vi "RSZVB Application Example.vi"(0 "VISA session":refnum<visa-resource-name>, 1 "Start Frequency (300.0e3 Hz)":dbl=300000.0 format="%^.3e", 2 "Power (0.0 dBm)":dbl format="%^.3e", 5 "Channel (1)":i32=1, 11 "error in (no error)":errorcluster {"code" format="%.0x"}, 12 "Stop Frequency (4.0e9 Hz)":dbl=4000000000.0 format="%^.3e") -> (4 "dup VISA session":refnum<visa-resource-name>, 6 "Stimulus Data":dbl[](array[numeric]) format="%^.3e", 8 "Response Data":dbl[](array[numeric]) format="%^.3e", 15 "error out":errorcluster {"code" format="%.0x"})   [LabVIEW 2011]
doc: "This VI is an simple example how to use instrument driver VIs."
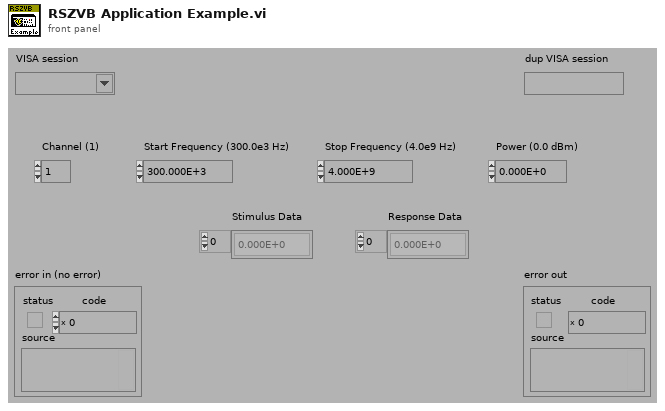
[diagram p1: front panel]
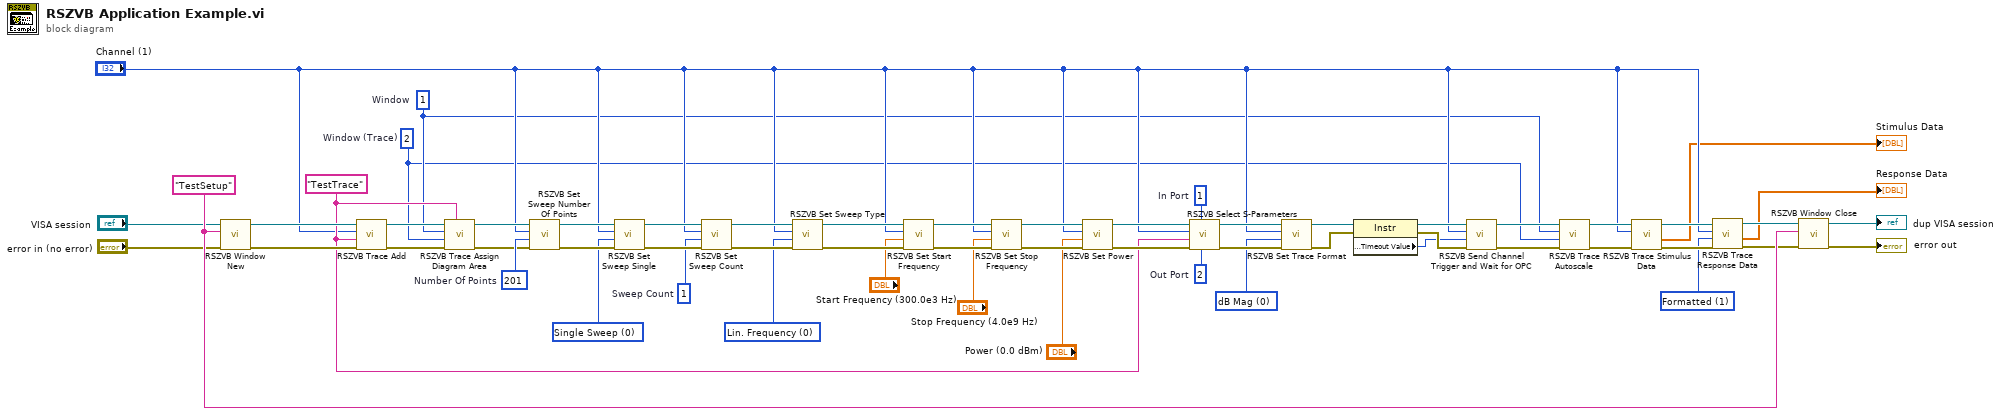
[diagram p0: block diagram]
diagram:
  w25 = 2  # Out Port
  w26 = 1  # In Port
  w6 = 2  # Window (Trace)
  w7 = 1  # Window
  w36 = 0 items=["dB Mag", "Phase", "Smith", "Polar", "Delay", "SWR", "Lin Mag", "Real", "Imag", "Inverted Smith", "Unwrapped Phase"] ("Format (0: dB Mag)")
  w39 = 1 items=["Unformatted", "Formatted"] ("Data Format (0: Unformatted)")
  w46 = 0 items=["Lin. Frequency", "Log. Frequency", "Segmented Frequency", "Power", "Time", "CW Mode"] ("Sweep Type (0: Lin. Frequency)")
  w49 = 201  # Number Of Points
  w50 = 1  # Sweep Count
  w51 = 0 items=["Single Sweep", "Continuous Sweep"] ("Single Sweep (1: Continuous Sweep)")
  w27 = "TestTrace" ("Trace Name (Trc1)")
  w24 = "TestSetup" ("Setup Name (Set1)")
  n1 = call "RSZVB Window New.vi"("error in (no error)"="error in (no error)", "Setup Name (Set1)"=w24, "VISA session"="VISA session") -> ("error out"=w57:errorcluster, "dup VISA session"=w56:refnum<visa-resource-name>)  [unwired: 7 in]
  n2 = call "RSZVB Trace Add.vi"("error in (no error)"=w57, "Trace Name (Trc1)"=w27, "Channel (1)"="Channel (1)", "VISA session"=w56) -> ("error out"=w30:errorcluster, "dup VISA session"=w31:refnum<visa-resource-name>)  [unwired: 6 in]
  n3 = call "RSZVB Trace Assign Diagram Area.vi"("Trace Name (Trc1)"=w27, "error in (no error)"=w30, "Window (Trace) (1)"=w6, "Window (1)"=w7, "VISA session"=w31) -> ("error out"=w28:errorcluster, "dup VISA session"=w29:refnum<visa-resource-name>)  [unwired: 5 in]
  n4 = call "RSZVB Set Sweep Number Of Points.vi"("error in (no error)"=w28, "Number Of Points (201)"=w49, "Channel (1)"="Channel (1)", "VISA session"=w29) -> ("error out"=w54:errorcluster, "dup VISA session"=w55:refnum<visa-resource-name>)  [unwired: 6 in]
  n5 = call "RSZVB Set Sweep Single.vi"("error in (no error)"=w54, "Single Sweep (1: Continuous Sweep)"=w51, "Channel (1)"="Channel (1)", "VISA session"=w55) -> ("error out"=w52:errorcluster, "dup VISA session"=w53:refnum<visa-resource-name>)  [unwired: 6 in]
  n6 = call "RSZVB Set Sweep Count.vi"("error in (no error)"=w52, "Sweep Count (1)"=w50, "Channel (1)"="Channel (1)", "VISA session"=w53) -> ("error out"=w47:errorcluster, "dup VISA session"=w48:refnum<visa-resource-name>)  [unwired: 6 in]
  n7 = call "RSZVB Set Sweep Type.vi"("error in (no error)"=w47, "Sweep Type (0: Lin. Frequency)"=w46, "Channel (1)"="Channel (1)", "VISA session"=w48) -> ("error out"=w44:errorcluster, "dup VISA session"=w45:refnum<visa-resource-name>)  [unwired: 6 in]
  n8 = call "RSZVB Set Start Frequency.vi"("error in (no error)"=w44, "Start Frequency (300.0e3 Hz)"="Start Frequency (300.0e3 Hz)", "Channel (1)"="Channel (1)", "VISA session"=w45) -> ("error out"=w14:errorcluster, "dup VISA session"=w15:refnum<visa-resource-name>)  [unwired: 6 in]
  n9 = call "RSZVB Set Stop Frequency.vi"("error in (no error)"=w14, "Stop Frequency (8.0e9 Hz)"="Stop Frequency (4.0e9 Hz)", "Channel (1)"="Channel (1)", "VISA session"=w15) -> ("error out"=w12:errorcluster, "dup VISA session"=w13:refnum<visa-resource-name>)  [unwired: 6 in]
  n10 = call "RSZVB Set Power.vi"("error in (no error)"=w12, "Power (0.0 dBm)"="Power (0.0 dBm)", "Channel (1)"="Channel (1)", "VISA session"=w13) -> ("error out"=w42:errorcluster, "dup VISA session"=w43:refnum<visa-resource-name>)  [unwired: 6 in]
  n11 = call "RSZVB Select S-Parameters.vi"("Out Port (1)"=w25, "In Port (1)"=w26, "error in (no error)"=w42, "Trace Name (Trc1)"=w27, "Channel (1)"="Channel (1)", "VISA session"=w43) -> ("error out"=w37:errorcluster, "dup VISA session"=w38:refnum<visa-resource-name>)  [unwired: 4 in]
  n12 = call "RSZVB Set Trace Format.vi"("error in (no error)"=w37, "Format (0: dB Mag)"=w36, "Channel (Trace) (1)"="Channel (1)", "VISA session"=w38) -> ("error out"=w34:errorcluster, "dup VISA session"=w35:refnum<visa-resource-name>)  [unwired: 6 in]
  n13 = property class="Instr"(reference=w35, error in=w34) -> (reference out=w23:refnum<visa-resource-name>, error out=w22:errorcluster, "General Settings:Timeout Value"=w19:u32)
  n14 = call "RSZVB Send Channel Trigger and Wait for OPC.vi"("error in (no error)"=w22, "Timeout (15000)"=w19, "Channel (1)"="Channel (1)", "VISA session"=w23) -> ("error out"=w21:errorcluster, "dup VISA session"=w20:refnum<visa-resource-name>)  [unwired: 6 in]
  n15 = call "RSZVB Trace Autoscale.vi"("error in (no error)"=w21, "Window (Trace) (1)"=w6, "Window (1)"=w7, "VISA session"=w20) -> ("error out"=w32:errorcluster, "dup VISA session"=w33:refnum<visa-resource-name>)  [unwired: 6 in]
  n16 = call "RSZVB Trace Stimulus Data.vi"("error in (no error)"=w32, "Channel (Trace) (1)"="Channel (1)", "VISA session"=w33) -> ("error out"=w40:errorcluster, "Trace Data"=→"Stimulus Data":dbl[], "dup VISA session"=w41:refnum<visa-resource-name>)  [unwired: 6 in]
  n17 = call "RSZVB Trace Response Data.vi"("error in (no error)"=w40, "Data Format (0: Unformatted)"=w39, "Channel (Trace) (1)"="Channel (1)", "VISA session"=w41) -> ("error out"=w16:errorcluster, "Trace Data"=→"Response Data":dbl[], "dup VISA session"=w17:refnum<visa-resource-name>)  [unwired: 5 in]
  n18 = call "RSZVB Window Close.vi"("error in (no error)"=w16, "Setup Name (Set1)"=w24, "VISA session"=w17) -> ("error out"=→"error out":errorcluster, "dup VISA session"=→"dup VISA session":refnum<visa-resource-name>)  [unwired: 7 in]
